vi "Extract Multiple Tone Information 1 Chan (CDB).vi"(0 "time signal in":waveform(cdb), 5 "export mode":T3(ring), 7 "threshold":dbl=0.001 format="%#_6p", 9 "max num tones":i32=4, 11 "error in (no error)":errorcluster, 12 "output sorting":i32(ring) items=["increasing frequency", "decreasing amplitude"]) -> (3 "exported signals":T1 {"exported spectrum (dB)"."dB Spectrum (Hann)" format="%.2p"; "exported spectrum (dB)"."df" format="%.2p"; "exported spectrum (dB)"."f0" format="%.2p"}, 4 "multiple tone information":T2(array[cluster]) {"detected phase (deg)" format="%_6g"; "detected amplitude" format="%_6p"; "detected frequency" format="%_6p"}, 15 "error out":errorcluster)   [LabVIEW 2020, in "NI_MAPro.lvlib"]
doc: "Returns the frequency, amplitude, and phase for each signal tone whose amplitude exceeds a specified <B>threshold</B>. Wire data to the <B>time signal in</B> input to determine the polymorphic instance to use or manually select the instance."
uses:
  NI_MAPro.lvlib
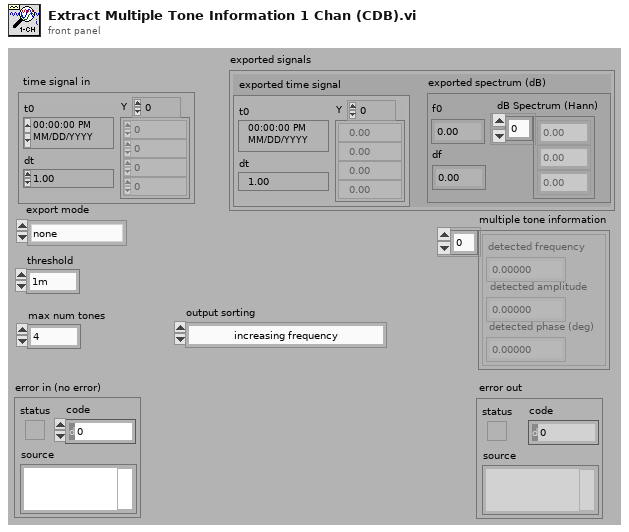
[diagram p1: front panel]
types:
  T1 = cluster{"exported time signal":waveform(cdb), "exported spectrum (dB)":cluster{"f0":dbl, "df":dbl, "dB Spectrum (Hann)":dbl[]}}
  T2 = cluster{"detected frequency":dbl, "detected amplitude":dbl, "detected phase (deg)":dbl}[]
  T3 = enum32{"none", "input signal", "detected signal", "residual signal"}
  T4 = typedef "NI_MAPro.lvlib/ma_sml_Spectral Info.ctl" = cluster{"spectrum type":enum16{"FFT Spectrum [complex]", "Amplitude [Magnitude]", "Power [Magnitude^2]", "Cross Spectrum [complex]", "Frequency Response [Complex]"}, "linear/dB":enum16{"linear", "dB"}, "window":u16, "window size":i32, "FFT size":i32}
  T5 = cluster{"Single/Multiple":enum16{"Multiple Peaks", "Single Max Peak"}, "threshold":dbl}
  T6 = cluster{"f0":dbl, "df":dbl, "complex Hann spectrum":cdb[]}
  T7 = typedef "NI_MAPro.lvlib/ma_sml_Spectrum Cluster (complex).ctl" = cluster{"f0":dbl, "df":dbl, "spectrum":cdb[]}
  T8 = cluster{"frequency":dbl, "amplitude":dbl, "phase [degree]":dbl}
  T9 = cluster{"frequency [Hz]":dbl, "amplitude":dbl, "phase [degree]":dbl}[]
  T10 = cluster{"time signal in":waveform(cdb), cluster{dbl, dbl, "Y":dbl[]}}
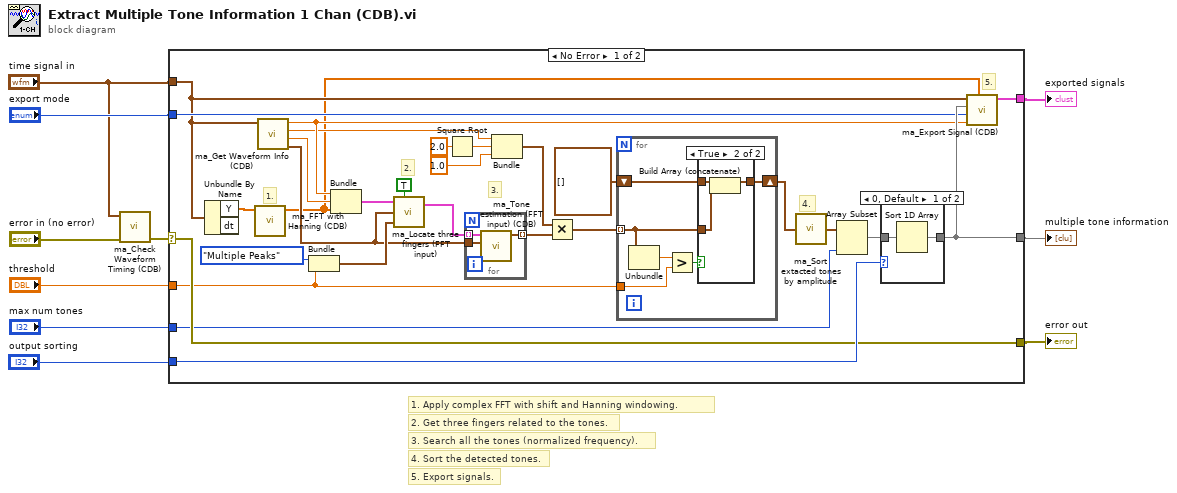
[diagram p0: block diagram]
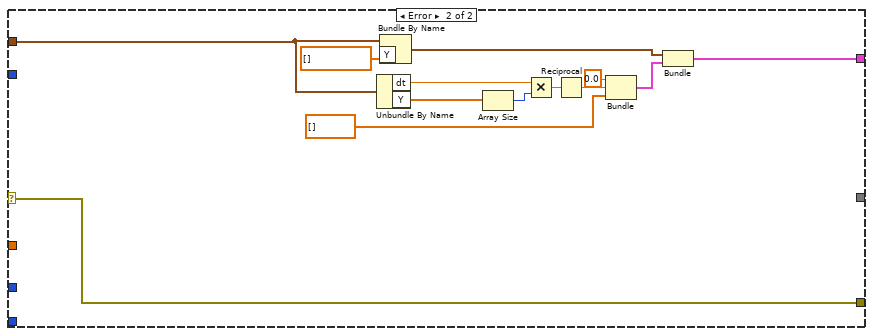
[diagram p4: hidden frame]
diagram:
  # "5. Export signals."
  # "4. Sort the detected tones."
  # "3. Search all the tones (normalized frequency)."
  # "2. Get three fingers related to the tones."
  # "1. Apply complex FFT with shift and Hanning windowing."
  n1 = call "ma_Check Waveform Timing (CDB).vi"("error in (no error)"="error in (no error)", "signal in"="time signal in") -> ("error out"=w7:errorcluster)  [unwired: 1 in, 8 out]
  n2 = case shown="No Error" w7 {
    selector: w7 -> [w29 w57]
    tunnel: [w24 _] -> w2
    tunnel: "threshold" -> [w11 _]
    tunnel: "max num tones" -> [w27 _]
    tunnel: "time signal in" -> [w21 w59]
    tunnel: [w22 w56] -> w1
    tunnel: "output sorting" -> [w30 _]
    tunnel: [w29 w57] -> w3
    tunnel: "export mode" -> [w23 _]
    frame No Error {
      # "5."
      # "3."
      # "4."
      # "2."
      # "1."
      n3 = Unbundle By Name(w21) -> ("Y"=w37:cdb[])  [unwired: 1 out]
      n4 = call "ma_FFT with Hanning (CDB).vi"("time signal data"=w37) -> ("complex Hann spectrum"=w15:cdb[])  [unwired: 10 out]
      n5 = call "ma_Get Waveform Info (CDB).vi"("time signal in"=w21) -> ("spectral info"=w18:T4, "df"=w17:dbl, "fs"=w16:dbl, "f0"=w20:dbl)  [unwired: 7 out]
      n6 = Bundle("Single/Multiple"=enum16{"Multiple Peaks", "Single Max Peak"}."Multiple Peaks", "threshold"=w11) -> (w31:T5)  [unwired: 1 out]
      n7 = Bundle("f0"=w20, "df"=w17, "complex Hann spectrum"=w15) -> (w39:T6)  [unwired: 1 out]
      n8 = call "ma_Locate three fingers (FFT input).vi"("spectrum includes end points?"=TRUE, "criterion"=w31, "spectral info"=w18, "FFT spectrum"=w39) -> ("three fingers (frequency normalized)"=w28:T7[])  [unwired: 1 out]
      n9 = Square Root(x=2.0) -> (sqrt(x)=w36:dbl)
      n10 = for {
        tunnel: w28 -> [w55] mode=indexing
        tunnel: w18 -> [w54]
        tunnel: [w53] -> w19 mode=indexing
        n11 = call "ma_Tone estimation (FFT input) (CDB).vi"("spectral info"=w54, "three fingers"=w55) -> ("single tone info."=w53:T8)  [unwired: 9 out]
      }
      n12 = Bundle("fs"=w16, w36, 1.0) -> (w33:cluster{"fs":dbl, dbl, dbl})  [unwired: 1 out]
      n13 = Multiply(x=w33, y=w19) -> (x*y=w13:cluster{dbl, dbl, dbl}[])
      n14 = for {
        tunnel: w13 -> [w42] mode=indexing
        tunnel: w11 -> [w45]
        shift-right: [w41] -> w12
        shift-left: cluster{dbl, dbl, dbl}[] [] -> [w40]
        n15 = Unbundle(w42) -> (w44:dbl)  [unwired: 2 out]
        n16 = Greater?(x=w44, y=w45) -> (0:w43:bool)
        n17 = case shown="True" w43 {
          tunnel: w42 -> [_ w48]
          tunnel: [w46 w47] -> w41
          tunnel: w40 -> [w46 w49]
          frame False {
          }
          frame True {
            n18 = Build Array (concatenate)(w49, w48) -> (w47:cluster{dbl, dbl, dbl}[])
          }
        }
      }
      n19 = call "ma_Sort extacted tones by amplitude.vi"("extracted tones in"=w12) -> ("extracted tones (sorted by amplitude)"=w26:T9)  [unwired: 4 out]
      n20 = Array Subset(array=w26, length=w27) -> (w25:T9)  [unwired: 1 in]
      n21 = case shown="0, Default" w30 {
        tunnel: w25 -> [w51 w52]
        tunnel: [w50 w52] -> w24
        frame 0, Default {
          n22 = Sort 1D Array(array=w51) -> (sorted array=w50:T9)
        }
        frame 1 {
        }
      }
      n23 = call "ma_Export Signal (CDB).vi"("complex Hann spectrum"=w15, "f0"=w20, "export signals"=w23, "multiple tone information"=w24, "time signal in"=w21) -> ("exported signals"=w22:T1)  [unwired: 1 in, 5 out]
    }
    frame Error {
      n24 = Unbundle By Name(w59) -> ("dt"=w66:dbl, "Y"=w64:cdb[])
      n25 = Bundle By Name(cluster=w59, "Y"=cdb[] []) -> (w60:waveform(cdb))
      n26 = Array Size(array=w64) -> (size(s)=w65:i32)
      n27 = Multiply(x=w66, y=w65) -> (x*y=w67:dbl)
      n28 = Reciprocal(x=w67) -> (1/x=w68:dbl)
      n29 = Bundle(0.0, w68, "Y"=dbl[] []) -> (w61:cluster{dbl, dbl, "Y":dbl[]})  [unwired: 1 out]
      n30 = Bundle("time signal in"=w60, w61) -> (w56:T10)  [unwired: 1 out]
    }
  }
  "multiple tone information" <- w2
  "exported signals" <- w1
  "error out" <- w3
